vi "Aero_Tunnel_Ph.vi"(8 "Target Speed":dbl caption="RPM" format="%.1f", 11 "Fan on Button":bool) -> ()   [LabVIEW 2010]
panel:
  in  "PitotZero button":bool
  in  "Stop HS Logging":bool
  in  "Start HS Logging":bool
  out "SmAD Data String":string
  out "Fan Running":bool
  out "Yaw Ready":bool caption="Ready"
  in  "Road on Button":bool
  out "P (mbar)":dbl caption="Current Setting" format="%.2f"
  in  "Set \"X\"Offset (mm)":dbl caption="0.000000" format="%.1f"
  in  "Quit":bool
  out "Road Ready":bool
  out "Road Fault":bool
  in  "Road Stop Button":bool
  out "Road Speed":dbl caption="m/s"
  in  "road speed selection":enum32{"road manual", "road sync to wind"}(radio)
  in  "Road target speed":dbl caption="Target  Speed" format="%.1f"
  in  "Road set speed  Button":bool caption="Set Speed"
  out "E-Stop Active":bool
  in  "Fan Stop button":bool
  out "Yaw Complete":bool caption="Complete"
  out "Yaw Limits":bool caption="Limits"
  out "Yaw Moving":bool caption="Moving"
  in  "yaw stop button":bool
  in  "Yaw GO Button":bool
  in  "Required Yaw":dbl format="%.2f"
  out "Yaw position":dbl(knob) caption="Degrees" scale=-5.0..5.0 scale format="%#_6f"
  in  "Update Balance Offsets":bool caption="V&H offsets"
  in  "Set \"Z\"Offset (mm)":dbl caption="0.000000" format="%.1f"
  in  "Data Net Button":bool
  in  "data ABS button":bool
  in  "SigConSetup":bool
  in  "Numeric Zero(All Axis) button":bool caption="Numeric Zero(All Axis)"
  in  "Boro Update":bool
  out "T (deg)":dbl caption="C"
  in  "P (mbar)":dbl caption="etting" format="%.2f"
  in  "E_STOP ALL":bool
  out "Fan Ready":bool
  out "Fan Speed":dbl caption="RPM"
  out "Wind Speed":dbl caption="m/s"
  in  "fan Set Speed":bool
  out "Roll gauge":dbl(slide) caption="100%             0                -100%" scale=-100.0..100.0
  out "Roll":dbl caption="N.m" format="%#.2f"
  out "Yaw gauge":dbl(slide) caption="100%             0                -100%" scale=-100.0..100.0
  out "Yaw":dbl caption="N.m" format="%#.2f"
  out "Side-force gauge":dbl(slide) caption="100%             0                -100%" scale=-100.0..100.0
  out "Side-Force":dbl caption="N" format="%#.2f"
  out "Drag Gauge":dbl(slide) caption="100%             0                -100%" scale=-100.0..100.0
  out "Drag":dbl caption="N" format="%#.2f"
  out "Pitch gauge":dbl(slide) caption="100%             0                -100%" scale=-100.0..100.0
  out "Pitch":dbl caption="N.m" format="%#.2f"
  out "Lift gauge":dbl(slide) caption="100%             0                -100%" scale=-100.0..100.0
  out "Lift":dbl caption="N" format="%#.2f"
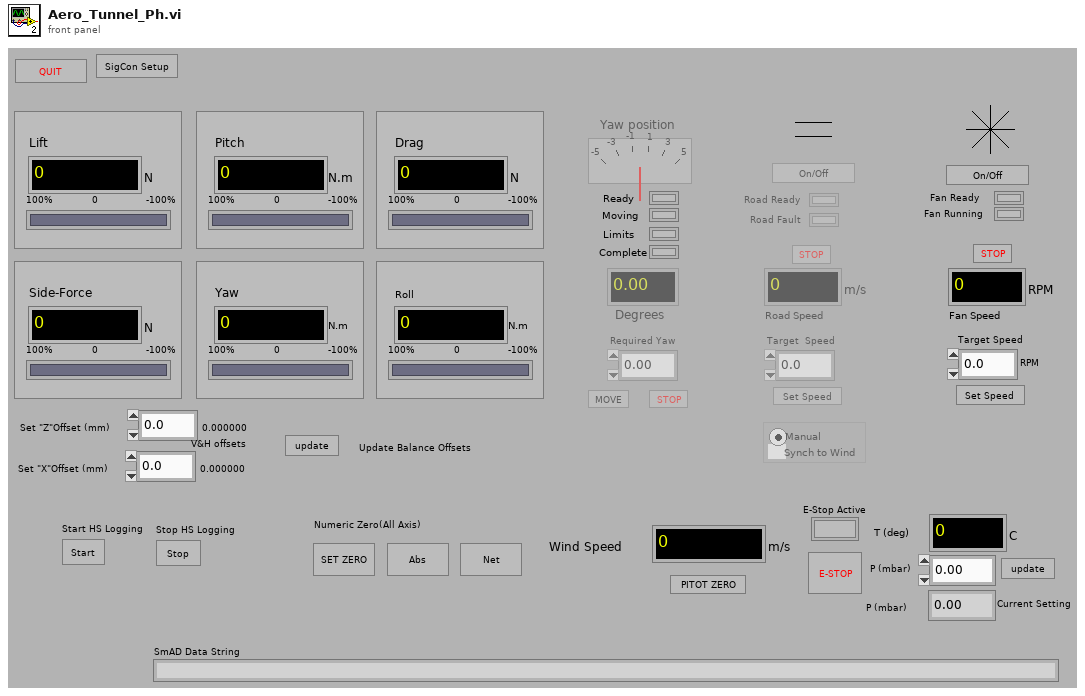
[diagram p1: front panel]
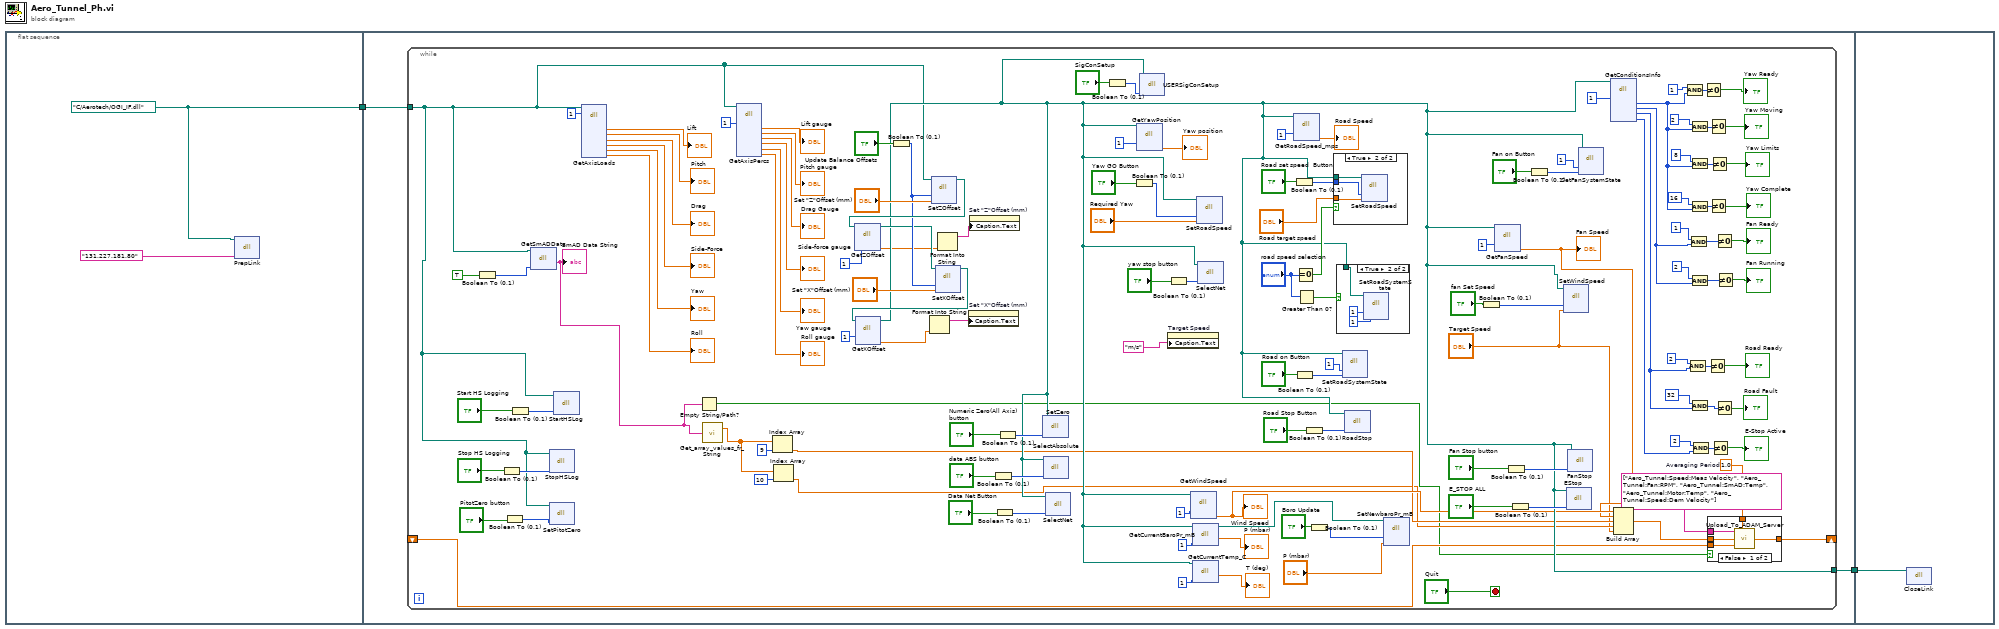
[diagram p0: block diagram]
diagram:
  n1 = flat-sequence {
    tunnel: [w4] -> w2
    tunnel: w2 -> [w6]
    tunnel: [w5] -> w1
    tunnel: w1 -> [w152]
    frame #0 {
      w4 = path "C:/Aerotech/OGI_IF.dll" ("path in")
      n2 = dll-call lib="C:/Aerotech/Drivers/OGI_IF.dll" fn="PrepLink"(path in=w4, "IPAddress"="131.227.181.80") -> ()  [unwired: 2 in, 4 out]
    }
    frame #1 {
      n3 = while {
        tunnel: w6 -> [w23]
        tunnel: [w41] -> w5
        shift-right: [w22] -> _
        shift-left: _ -> [w21]
        stop <- "Quit" stop-if-true
        w19 = 1.0  # Averaging Period
        n4 = Boolean To (0,1)(Boolean=TRUE) -> (0, 1=w30:i16)
        n5 = Boolean To (0,1)(Boolean="Stop HS Logging") -> (0, 1=w26:i16)
        n6 = Boolean To (0,1)(Boolean="PitotZero button") -> (0, 1=w24:i16)
        n7 = Boolean To (0,1)(Boolean="Start HS Logging") -> (0, 1=w29:i16)
        n8 = dll-call lib="C:/Aerotech/Drivers/OGI_IF.dll" fn="GetSmADData"(path in=w23, "Enable"=w30) -> ("SmAD Data String"=w8:string)  [unwired: 2 in, 3 out]
        "SmAD Data String" <- w8
        n9 = dll-call lib="C:/Aerotech/Drivers/OGI_IF.dll" fn="StopHSLog"(path in=w23, "Enable"=w26) -> ()  [unwired: 2 in, 4 out]
        n10 = dll-call lib="C:/Aerotech/Drivers/OGI_IF.dll" fn="SetPitotZero"(path in=w23, "Enable"=w24) -> ()  [unwired: 2 in, 4 out]
        n11 = dll-call lib="C:/Aerotech/Drivers/OGI_IF.dll" fn="StartHSLog"(path in=w23, "Enable"=w29) -> ()  [unwired: 2 in, 4 out]
        n12 = dll-call lib="C:/Aerotech/Drivers/OGI_IF.dll" fn="GetAxisLoads"(path in=w23, "Enable"=1) -> ("Lift"=→"Lift":dbl, "Pitch"=→"Pitch":dbl, "Drag"=→"Drag":dbl, "side"=→"Side-Force":dbl, "Yaw"=→"Yaw":dbl, "Roll"=→"Roll":dbl)  [unwired: 3 in, 9 out]
        n13 = Empty String/Path?(string/path=w8) -> (empty?=w7:bool)
        n14 = call "Get_array_values_fr_String.vi"("String Value"=w8) -> ("Numeric Array"=w12:dbl[])  [unwired: 1 out]
        n15 = dll-call lib="C:/Aerotech/Drivers/OGI_IF.dll" fn="GetAxisPercs"(path in=w23, "Enable"=1) -> ("Lift"=→"Lift gauge":dbl, "Pitch"=→"Pitch gauge":dbl, "Drag"=→"Drag Gauge":dbl, "side"=→"Side-force gauge":dbl, "Yaw"=→"Yaw gauge":dbl, "Roll"=→"Roll gauge":dbl)  [unwired: 3 in, 9 out]
        n16 = Index Array(array=w12, index=9) -> (element=w11:dbl)
        n17 = Index Array(array=w12, index=10) -> (element=w10:dbl)
        n18 = Boolean To (0,1)(Boolean="Update Balance Offsets") -> (0, 1=w123:i16)
        n19 = dll-call lib="C:/Aerotech/Drivers/OGI_IF.dll" fn="SetZOffset"(path in=w23, "Enable"=w123, "SetZoffset"="Set \"Z\"Offset (mm)") -> (path out=w124:path)  [unwired: 3 in, 3 out]
        n20 = dll-call lib="C:/Aerotech/Drivers/OGI_IF.dll" fn="GetZOffset"(path in=w124, "Enable"=1) -> (path out=w120:path, "ZOffset"=w38:dbl)  [unwired: 3 in, 3 out]
        n21 = dll-call lib="C:/Aerotech/Drivers/OGI_IF.dll" fn="SetXOffset"(path in=w120, "Enable"=w123, "SetXOffset"="Set \"X\"Offset (mm)") -> (path out=w119:path)  [unwired: 3 in, 3 out]
        n22 = dll-call lib="C:/Aerotech/Drivers/OGI_IF.dll" fn="GetXOffset"(path in=w119, "Enable"=1) -> (path out=w41:path, "XOffset"=w36:dbl)  [unwired: 3 in, 3 out]
        n23 = Format Into String(w36) -> (resulting string=w122:string)  [unwired: 3 in, 1 out]
        n24 = Format Into String(w38) -> (resulting string=w37:string)  [unwired: 3 in, 1 out]
        n25 = property on="Set \"X\"Offset (mm)" class="DigNum (strict)"("Caption.Text"=w122) -> ()  [unwired: 2 in, 2 out]
        n26 = property on="Set \"Z\"Offset (mm)" class="DigNum (strict)"("Caption.Text"=w37) -> ()  [unwired: 2 in, 2 out]
        n27 = Boolean To (0,1)(Boolean="data ABS button") -> (0, 1=w111:i16)
        n28 = Boolean To (0,1)(Boolean="Data Net Button") -> (0, 1=w114:i16)
        n29 = Boolean To (0,1)(Boolean="Numeric Zero(All Axis) button") -> (0, 1=w117:i16)
        n30 = dll-call lib="C:/Aerotech/Drivers/OGI_IF.dll" fn="SetZero"(path in=w41, "Enable"=w117) -> ()  [unwired: 2 in, 4 out]
        n31 = dll-call lib="C:/Aerotech/Drivers/OGI_IF.dll" fn="SelectAbsolute"(path in=w41, "Enable"=w111) -> ()  [unwired: 2 in, 4 out]
        n32 = dll-call lib="C:/Aerotech/Drivers/OGI_IF.dll" fn="SelectNet"(path in=w41, "Enable"=w114) -> ()  [unwired: 2 in, 4 out]
        n33 = Boolean To (0,1)(Boolean="SigConSetup") -> (0, 1=w104:i16)
        n34 = Boolean To (0,1)(Boolean="Yaw GO Button") -> (0, 1=w40:i16)
        n35 = dll-call lib="C:/Aerotech/Drivers/OGI_IF.dll" fn="GetYawPosition"(path in=w41, "Enable"=1) -> ("YawPosDeg"=→"Yaw position":dbl)  [unwired: 3 in, 4 out]
        n36 = dll-call lib="C:/Aerotech/Drivers/OGI_IF.dll" fn="USERSigConSetup"(path in=w41, "Enable"=w104) -> ()  [unwired: 2 in, 4 out]
        n37 = property on="Target Speed" class="DigNum (strict)"("Caption.Text"="m/s") -> ()  [unwired: 2 in, 2 out]
        n38 = Boolean To (0,1)(Boolean="yaw stop button") -> (0, 1=w79:i16)
        n39 = dll-call lib="C:/Aerotech/Drivers/OGI_IF.dll" fn="GetWindSpeed"(path in=w41, "Enable"=1) -> ("Windspeed_M/s"=w18:dbl)  [unwired: 3 in, 4 out]
        "Wind Speed" <- w18
        n40 = dll-call lib="C:/Aerotech/Drivers/OGI_IF.dll" fn="GetCurrentBaroPr_mB"(path in=w41, "Enable"=1) -> (path out=w33:path, "mbar"=→"P (mbar)":dbl)  [unwired: 3 in, 1 out]
        n41 = dll-call lib="C:/Aerotech/Drivers/OGI_IF.dll" fn="GetCurrentTemp_C"(path in=w41, "Enable"=1) -> ("Deg_C"=→"T (deg)":dbl)  [unwired: 3 in, 2 out]
        n42 = dll-call lib="C:/Aerotech/Drivers/OGI_IF.dll" fn="SetRoadSpeed"(path in=w41, "Enable"=w40, "NewRoadSpeed"="Required Yaw") -> ()  [unwired: 2 in, 5 out]
        n43 = dll-call lib="C:/Aerotech/Drivers/OGI_IF.dll" fn="SelectNet"(path in=w41, "Enable"=w79) -> ()  [unwired: 2 in, 4 out]
        n44 = dll-call lib="C:/Aerotech/Drivers/OGI_IF.dll" fn="GetRoadSpeed_mps"(path in=w41, "Enable"=1) -> ("RoadSpeedm/s"=→"Road Speed":dbl)  [unwired: 3 in, 4 out]
        n45 = Boolean To (0,1)(Boolean="Road set speed  Button") -> (0, 1=w91:i16)
        n46 = Boolean To (0,1)(Boolean="Road on Button") -> (0, 1=w85:i16)
        n47 = Equal To 0?(x="road speed selection") -> (x = 0?=w93:bool)
        n48 = Greater Than 0?(x="road speed selection") -> (x > 0?=w88:bool)
        n49 = Boolean To (0,1)(Boolean="Road Stop Button") -> (0, 1=w83:i16)
        n50 = Boolean To (0,1)(Boolean="Boro Update") -> (0, 1=w32:i16)
        n51 = case shown="True" w93 {
          tunnel: w41 -> [_ w151]
          tunnel: w91 -> [_ w150]
          tunnel: "Road target speed" -> [_ w149]
          frame False {
          }
          frame True {
            n52 = dll-call lib="C:/Aerotech/Drivers/OGI_IF.dll" fn="SetRoadSpeed"(path in=w151, "Enable"=w150, "NewRoadSpeed"=w149) -> ()  [unwired: 3 in, 4 out]
          }
        }
        n53 = case shown="True" w88 {
          tunnel: w41 -> [_ w146]
          frame False {
          }
          frame True {
            n54 = dll-call lib="C:/Aerotech/Drivers/OGI_IF.dll" fn="SetRoadSystemState"(path in=w146, "Enable"=1, "RoadSyncToWind"=1) -> ()  [unwired: 4 in, 3 out]
          }
        }
        n55 = dll-call lib="C:/Aerotech/Drivers/OGI_IF.dll" fn="SetRoadSystemState"(path in=w41, "Enable"=1, "Road ONOFF"=w85) -> ()  [unwired: 3 in, 4 out]
        n56 = dll-call lib="C:/Aerotech/Drivers/OGI_IF.dll" fn="RoadStop"(path in=w41, "Enable"=w83) -> ()  [unwired: 2 in, 4 out]
        n57 = dll-call lib="C:/Aerotech/Drivers/OGI_IF.dll" fn="SetNewbaroPr_mB"(path in=w33, "Enable"=w32, "NewPressure"="P (mbar)") -> ()  [unwired: 3 in, 4 out]
        n58 = Boolean To (0,1)(Boolean="fan Set Speed") -> (0, 1=w43:i16)
        n59 = dll-call lib="C:/Aerotech/Drivers/OGI_IF.dll" fn="GetFanSpeed"(path in=w41, "Enable"=1) -> ("FanSpeedinRPM"=w17:dbl)  [unwired: 3 in, 4 out]
        "Fan Speed" <- w17
        n60 = Boolean To (0,1)(Boolean="Fan Stop button") -> (0, 1=w109:i16)
        n61 = Boolean To (0,1)(Boolean="E_STOP ALL") -> (0, 1=w97:i16)
        n62 = Boolean To (0,1)(Boolean="Fan on Button") -> (0, 1=w77:i16)
        n63 = dll-call lib="C:/Aerotech/Drivers/OGI_IF.dll" fn="SetWindSpeed"(path in=w41, "Enable"=w43, "NewWindSpeed"="Target Speed") -> ()  [unwired: 3 in, 4 out]
        n64 = dll-call lib="C:/Aerotech/Drivers/OGI_IF.dll" fn="EStop"(path in=w41, "Enable"=w97) -> ()  [unwired: 2 in, 4 out]
        n65 = dll-call lib="C:/Aerotech/Drivers/OGI_IF.dll" fn="FanStop"(path in=w41, "Enable"=w109) -> ()  [unwired: 2 in, 4 out]
        n66 = dll-call lib="C:/Aerotech/Drivers/OGI_IF.dll" fn="SetFanSystemState"(path in=w41, "Enable"=1, "Fan ONOFF"=w77) -> ()  [unwired: 3 in, 4 out]
        n67 = dll-call lib="C:/Aerotech/Drivers/OGI_IF.dll" fn="GetConditionsInfo"(path in=w41, "Enable"=1) -> ("YawControl"=w56:i32, "FanControl"=w44:i32, "RoadControl"=w55:i32, "Globals"=w51:i32)  [unwired: 3 in, 7 out]
        n68 = Build Array(w18, w17, w11, w10, "Target Speed") -> (w16:dbl[])
        n69 = Compound Arithmetic op=AND(1 ("value"), w56) -> (w76:i32)
        n70 = Compound Arithmetic op=AND(2 ("value"), w55) -> (w60:i32)
        n71 = Compound Arithmetic op=AND(1 ("value"), w44) -> (w64:i32)
        n72 = Compound Arithmetic op=AND(2 ("value"), w56) -> (w73:i32)
        n73 = Compound Arithmetic op=AND(16 ("value"), w56) -> (w71:i32)
        n74 = Compound Arithmetic op=AND(2 ("value"), w44) -> (w45:i32)
        n75 = Compound Arithmetic op=AND(8 ("value"), w56) -> (w72:i32)
        n76 = Compound Arithmetic op=AND(32 ("value"), w55) -> (w59:i32)
        n77 = Compound Arithmetic op=AND(2 ("value"), w51) -> (w54:i32)
        n78 = Not Equal To 0?(x=w76) -> (x != 0?=→"Yaw Ready":bool)
        n79 = Not Equal To 0?(x=w60) -> (x != 0?=→"Road Ready":bool)
        n80 = case shown="False" w7 {
          tunnel: [w144 w145] -> w22
          tunnel: w21 -> [w143 w145]
          tunnel: string[] ["Aero_Tunnel:Speed:Meas Velocity", "Aero_Tunnel:Fan:RPM", "Aero_Tunnel:SmAD:Temp", "Aero_Tunnel:Motor:Temp", "Aero_Tunnel:Speed:Dem Velocity"] ("Channel Names") -> [w142 _]
          tunnel: w19 -> [w141 _]
          tunnel: w16 -> [w140 _]
          frame False {
            n81 = call "Upload_To_ADAM_Server.vi"("Channel Names"=w142, "Averaging Period (s)"=w141, "Channel Values"=w140, "Shift In"=w143) -> ("Shift Out"=w144:dbl[])  [unwired: 1 out]
          }
          frame True {
          }
        }
        n82 = Not Equal To 0?(x=w73) -> (x != 0?=→"Yaw Moving":bool)
        n83 = Not Equal To 0?(x=w71) -> (x != 0?=→"Yaw Complete":bool)
        n84 = Not Equal To 0?(x=w72) -> (x != 0?=→"Yaw Limits":bool)
        n85 = Not Equal To 0?(x=w54) -> (x != 0?=→"E-Stop Active":bool)
        n86 = Not Equal To 0?(x=w59) -> (x != 0?=→"Road Fault":bool)
        n87 = Not Equal To 0?(x=w64) -> (x != 0?=→"Fan Ready":bool)
        n88 = Not Equal To 0?(x=w45) -> (x != 0?=→"Fan Running":bool)
      }
    }
    frame #2 {
      n89 = dll-call lib="C:/Aerotech/Drivers/OGI_IF.dll" fn="CloseLink"(path in=w152) -> ()  [unwired: 2 in, 3 out]
    }
  }
